vi "Intake deal with joysticks.vi"(1 "Extend?":bool, 2 "Negative Throttle (%)":dbl, 3 "Positive Throttle (%)":dbl) -> (0 "Intake Teleop Command":T1)   [LabVIEW 2019]
uses:
  Intake Command Type Def.ctl
  Intake Mode Type Def.ctl
  <vilib>/Rock Robotics/WPI/Solenoid/WPI_SolenoidValue.ctl
panel:
  # "INTAKE AUTO-EXTENDS / RETRACTS IF TRIGGERS PRESSED >75%\nOtherwise stays at prior state"
  # "Positive is IN\nNEGATIVE IS OUT"
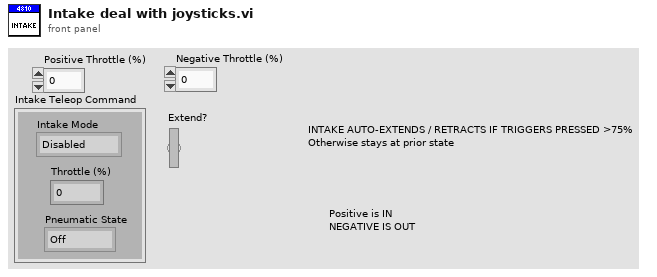
[diagram p1: front panel]
types:
  T1 = typedef "Intake Command Type Def.ctl" = cluster{"Intake Mode":T2, "Throttle (%)":dbl, "Pneumatic State":T3}
  T2 = typedef "Intake Mode Type Def.ctl" = enum16{"Disabled", "Enabled"}
  T3 = typedef "WPI_SolenoidValue.ctl" = enum16{"Off", "On", "Forward", "Reverse"}
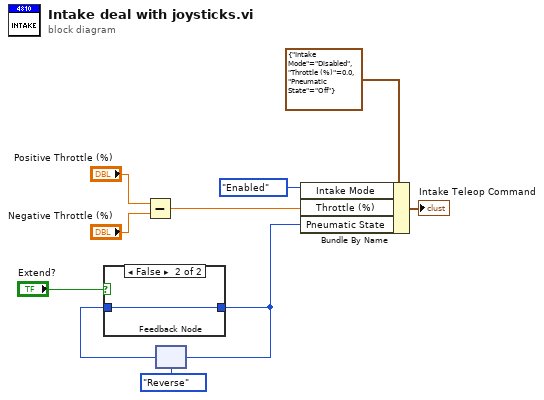
[diagram p0: block diagram]
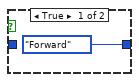
[diagram p2: hidden frame]
diagram:
  n1 = Subtract(x="Positive Throttle (%)", y="Negative Throttle (%)") -> (x-y=w5:dbl)
  n2 = feedback #1(WPI_SolenoidValue."Reverse" ("Pneumatic State")) -> (w4:T3)
  n3 = case shown="False" "Extend?" {
    tunnel: [WPI_SolenoidValue."Forward" ("Pneumatic State") w12] -> w2
    tunnel: w4 -> [_ w12]
    frame True {
    }
    frame False {
    }
  }
  n4 = feedback-in #1(w2) -> ()
  n5 = Bundle By Name(cluster=T1 {"Intake Mode"=enum."Disabled", "Throttle (%)"=0.0, "Pneumatic State"=enum."Off"} ("Teleop Intake Command"), "Intake Mode"=Intake_Mode_Type_Def."Enabled", "Throttle (%)"=w5, "Pneumatic State"=w2) -> (→"Intake Teleop Command":T1)
